vi "Initialize.vi"(8 "error in":errorcluster, 11 "Plugin in":refnum<class "DateTimeChannel.lvclass">) -> (0 "error out":errorcluster, 3 "Plugin out":refnum<class "DateTimeChannel.lvclass">)   [LabVIEW 2023, in "DateTimeChannel.lvlib" / "DateTimeChannel.lvclass"]
uses:
  DateTimeChannel.lvclass
  C:/Program Files/National Instruments/LabVIEW 2023/vi.lib/FlexLogger/SDK/PluginSDK.lvlibp/PEFClasses/SDK/Plugin/Plugin.lvclass
  <vilib>/FlexLogger/SDK/PluginSDK.lvlibp/PEFClasses/SDK/Processing Element/Timing Parameters.ctl
  <vilib>/FlexLogger/SDK/PluginSDK.lvlibp/PEFClasses/SDK/Processing Element/Timing Method.ctl
  <vilib>/FlexLogger/SDK/PluginSDK.lvlibp/PEFClasses/SDK/Channel/Data Type_v2.ctl
  <vilib>/FlexLogger/SDK/PluginSDK.lvlibp/PEFClasses/SDK/Producer Channel/Producer Channel.lvclass
  C:/Program Files/National Instruments/LabVIEW 2023/vi.lib/FlexLogger/SDK/PluginSDK.lvlibp/PEFClasses/SDK/Channel/Channel.lvclass
  <vilib>/FlexLogger/SDK/PluginSDK.lvlibp/PEFClasses/SDK/Plugin/ParameterAccess/Write String.vi
  <vilib>/FlexLogger/SDK/PluginSDK.lvlibp/PEFClasses/SDK/Producer Channel/Create Producer Channel_v2.vi
  <vilib>/FlexLogger/SDK/PluginSDK.lvlibp/PEFClasses/SDK/Plugin/Plugin.lvclass
  <vilib>/FlexLogger/SDK/PluginSDK.lvlibp/PEFClasses/SDK/Processing Element/Processing Element.lvclass
  C:/Program Files/National Instruments/LabVIEW 2023/vi.lib/FlexLogger/SDK/PluginSDK.lvlibp/PEFClasses/SDK/Processing Element/Processing Element.lvclass
  C:/Users/bbuchana/Documents/LabVIEW Projects/FlexLogger IO Plug-ins/DateTimeChannel/DateTimeChannel.lvclass
  <vilib>/FlexLogger/SDK/PluginSDK.lvlibp
  <vilib>/FlexLogger/SDK/PluginSDK.lvlibp/PEFClasses/SDK/Channel/Channel.lvclass
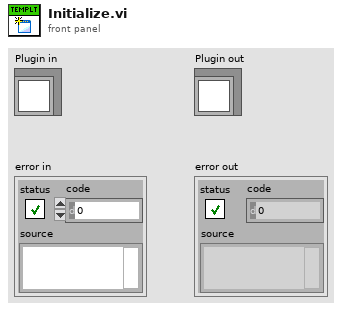
[diagram p1: front panel]
types:
  T1 = typedef "PluginSDK.lvlibp/Channel.lvclass/Data Type_v2.ctl" = u16
  T2 = typedef "PluginSDK.lvlibp/Processing Element.lvclass/Timing Parameters.ctl" = cluster{"Timing Method":T3, "Timing Period (ms)":i32}
  T3 = typedef "PluginSDK.lvlibp/Processing Element.lvclass/Timing Method.ctl" = enum16{"Periodic", "Immediate", "On Data Ready", "Triggered"}
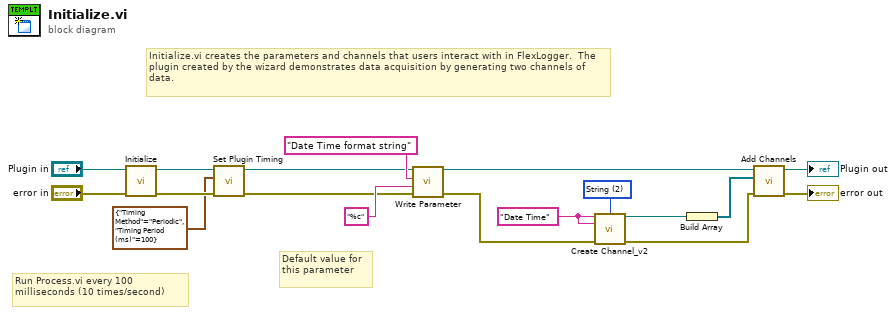
[diagram p0: block diagram]
diagram:
  w4 = "Date Time" ("Unique Channel Identifier")
  w5 = T1 2 items=["Wfm (DBL)", "Wfm (Digital)", "String"] ("Data Type")
  # "Default value for this parameter"
  # "Run Process.vi every 100 milliseconds (10 times/second)"
  # "Initialize.vi creates the parameters and channels that users interact with in FlexLogger.  The plugin created by the wizard demonstrates data acquisition by generating two channels of data."
  n1 = call-parent "Initialize.vi"("error in (no error)"="error in", "Plugin in"="Plugin in") -> ("error out"=w12:errorcluster, "Plugin out"=w10:refnum<class "DateTimeChannel.lvclass">)  [unwired: 8 in]
  n2 = call <vilib>:"Set Plugin Timing.vi"("error in (no error)"=w12, "Timing Parameters"=T2 {"Timing Method"=enum."Periodic", "Timing Period (ms)"=100}, "Plugin in"=w10) -> ("error out"=w8:errorcluster, "Plugin out"=w9:refnum<class "DateTimeChannel.lvclass">)  [unwired: 7 in]
  n3 = call-poly <vilib>:"Write Parameter.vi"("error in (no error)"=w8, "Value"="%c", "Name"="Date Time format string", "Plugin in"=w9) -> ("error out"=w6:errorcluster, "Plugin out"=w7:refnum<class "DateTimeChannel.lvclass">)  [unwired: 6 in]
  n4 = call-poly <vilib>:"Create Channel_v2.vi"("Unique Channel Identifier"=w4, "Data Type"=w5, "Default Channel Name"=w4, "error in (no error)"=w6) -> ("Producer Channel"=w3:refnum<class "Producer Channel.lvclass">, "error out"=w1:errorcluster)  [unwired: 10 in]
  n5 = Build Array(w3) -> (w2:refnum<class "Producer Channel.lvclass">[])
  n6 = call <vilib>:"Add Channels.vi"("error in (no error)"=w1, "Channels"=w2, "Plugin in"=w7) -> ("error out"=→"error out":errorcluster, "Plugin out"=→"Plugin out":refnum<class "DateTimeChannel.lvclass">)  [unwired: 7 in]
